vi "探测器列表-登记新设备.vi"(6 "探测器信息":T1, 7 "table-探测器列表名":string="探测器列表", 8 "error in (no error)":errorcluster, 9 "元素名[]-探测器信息":string[](array[string]), 11 "数据库引用":T4) -> (0 "error out":errorcluster, 3 "connection reference out":T4)   [LabVIEW 2017]
doc: "添加新设备 , 并且新建数据表 ."
uses:
  <vilib>/addons/database/Connection.llb/Conn ObjectReference.ctl
  <vilib>/addons/database/Auxilliary.llb/DB Tools Column Info.ctl
  <vilib>/addons/database/Auxilliary.llb/DB Tools DataTypes.ctl
  <vilib>/addons/database/NI_Database_API.lvlib
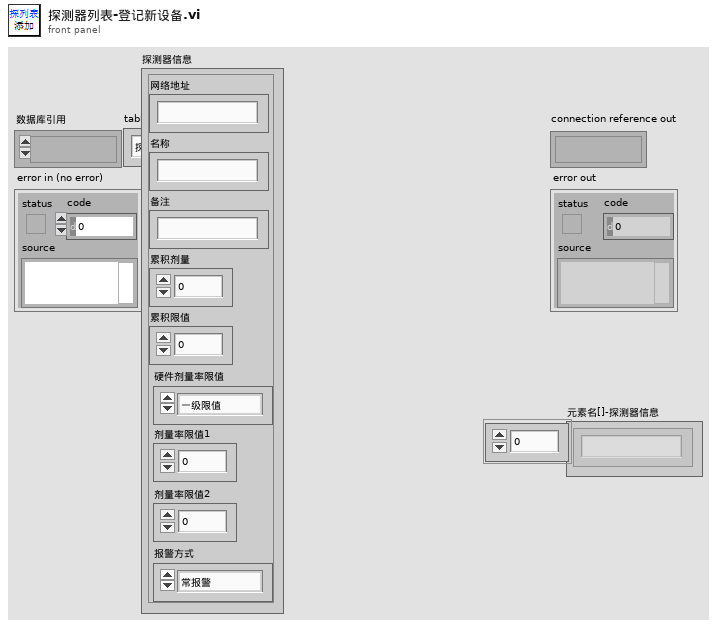
[diagram p1: front panel]
types:
  T1 = typedef "探测器信息.ctl" = cluster{"网络地址":string, "名称":string, "备注":string, "累积剂量":dbl, "累积限值":dbl, "硬件剂量率限值":T2, "剂量率限值1":dbl, "剂量率限值2":dbl, "报警方式":T3}
  T2 = typedef "探头剂量率限值选择.ctl" = enum16{"一级限值", "二级限值"}
  T3 = typedef "报警方式选择.ctl" = enum16{"常报警", "自动静音", "手动静音"}
  T4 = typedef "NI_Database_API.lvlib/Conn ObjectReference.ctl" = refnum<k1>
  T5 = typedef "NI_Database_API.lvlib/DB Tools Column Info.ctl" = cluster{"column name":string, "data type":T6, "size":i32, "allow null?":bool}
  T6 = typedef "NI_Database_API.lvlib/DB Tools DataTypes.ctl" = enum16{"String", "Long (I32)", "Single (SGL)", "Double (DBL)", "Date/Time", "Binary"}
  T7 = typedef "单条累积记录.ctl" = cluster{"起始时间":timestamp, "结束时间":timestamp, "累积剂量":dbl}
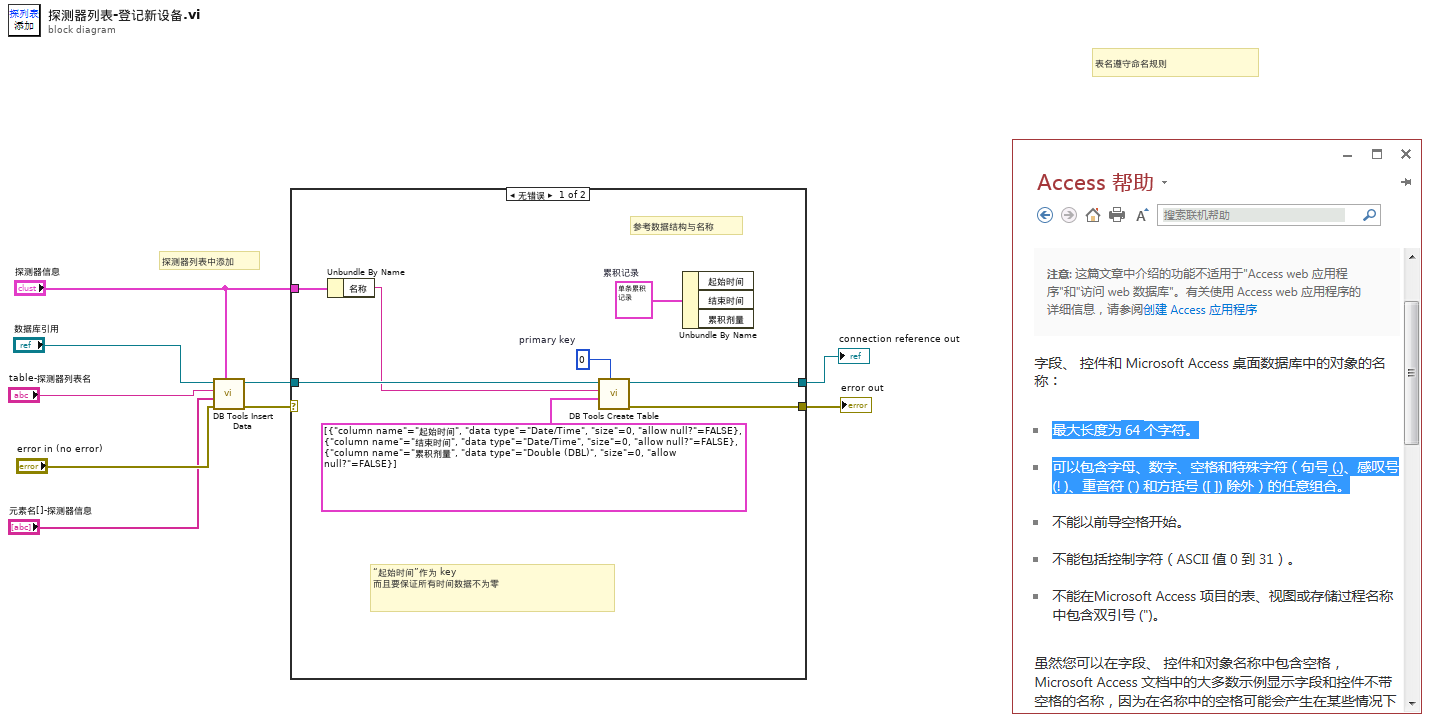
[diagram p0: block diagram]
diagram:
  # "表名遵守命名规则"
  # "探测器列表中添加"
  n1 = call <vilib>:"DB Tools Insert Data.vi"("data"="探测器信息", "error in (no error)"="error in (no error)", "columns"="元素名[]-探测器信息", "table"="table-探测器列表名", "connection reference"="数据库引用") -> ("error out"=w5:errorcluster, "connection reference out"=w4:T4)  [unwired: 5 in]
  n2 = case shown="无错误" w5 {
    selector: w5 -> [_ w18]
    tunnel: w4 -> [w15 w19]
    tunnel: "探测器信息" -> [w14 _]
    tunnel: [w12 w18] -> w2
    tunnel: [w11 w19] -> w1
    frame No Error {
      w10 = T7 {"起始时间"=timestamp(0 s since 1904-01-01), "结束时间"=timestamp(0 s since 1904-01-01), "累积剂量"=0.0}  # 累积记录
      w17 = 0  # primary key
      # "参考数据结构与名称"
      # "“起始时间”作为 key\n而且要保证所有时间数据不为零"
      n3 = Unbundle By Name(w14) -> ("名称"=w13:string)
      n4 = call <vilib>:"DB Tools Create Table.vi"("primary key (-1)"=w17, "column information"=T5[] [{"column name"="起始时间", "data type"=enum."Date/Time", "size"=0, "allow null?"=FALSE}, {"column name"="结束时间", "data type"=enum."Date/Time", "size"=0, "allow null?"=FALSE}, {"column name"="累积剂量", "data type"=enum."Double (DBL)", "size"=0, "allow null?"=FALSE}], "table"=w13, "connection reference"=w15) -> ("error out"=w12:errorcluster, "connection reference out"=w11:T4)  [unwired: 4 in]
      n5 = Unbundle By Name(w10) -> ()  [unwired: 3 out]
    }
    frame Error {
    }
  }
  "connection reference out" <- w1
  "error out" <- w2
